vi "IDS_ecu_getParameters.vi"(8 "error in (no error)":errorcluster, 11 "deviceHandle":i32) -> (0 "error out":errorcluster, 2 "ECU parameters":T1, 3 "deviceHandle out":i32)   [LabVIEW 2016]
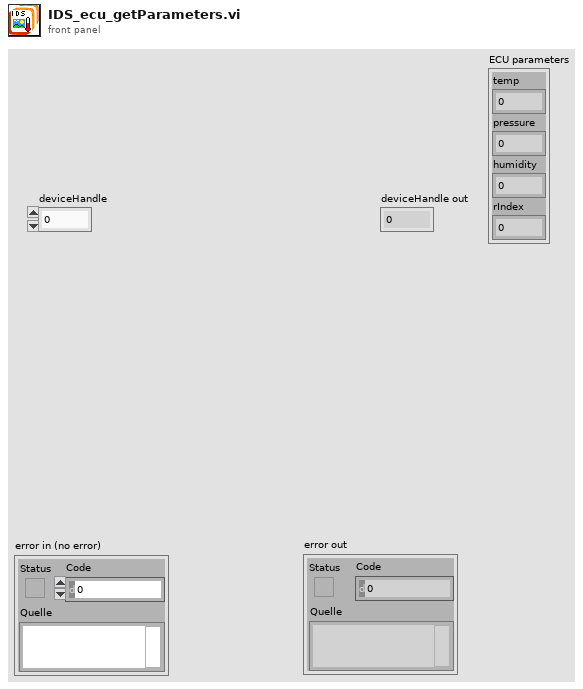
[diagram p1: front panel]
types:
  T1 = cluster{"temp":dbl, "pressure":dbl, "humidity":dbl, "rIndex":dbl}
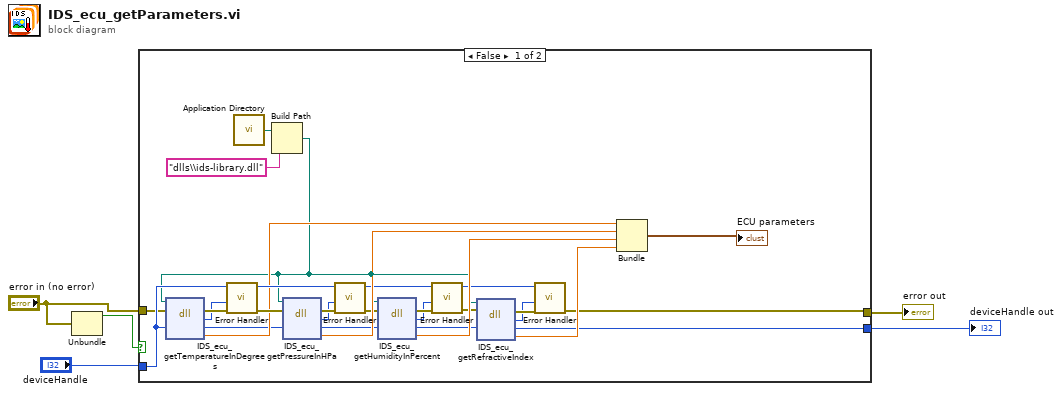
[diagram p0: block diagram]
diagram:
  n1 = Unbundle("error in (no error)") -> ("status"=w2:bool)  [unwired: 2 out]
  n2 = case shown="False" w2 {
    tunnel: [w10 w36] -> w5
    tunnel: [w11 w35] -> w4
    tunnel: "deviceHandle" -> [w20 w35]
    tunnel: "error in (no error)" -> [w14 w36]
    frame False {
      n3 = call <vilib>:"Application Directory.vi"() -> ("Application Directory"=w8:path)
      n4 = Build Path(base path=w8, name or relative path="dlls\\ids-library.dll" ("ipAddress")) -> (appended path=w6:path)
      n5 = dll-call lib="C:/Users/matheus/Desktop/LabVIEW_Draft_V1.6.0/dlls/ids-library.*" fn="IDS_ecu_getTemperatureInDegrees"(path in=w6, error in=w14, "deviceHandle"=w20) -> (error out=w31:errorcluster, "return type"=w24:i32, "deviceHandle"=w12:i32, "temp"=w13:dbl)  [unwired: 2 in, 1 out]
      n6 = call "Error Handler.vi"("error in (no error)"=w31, "error code"=w24, "deviceHandle"=w20) -> ("error out"=w30:errorcluster, "deviceHandle Out"=w17:i32)  [unwired: 7 in]
      n7 = dll-call lib="C:/Users/matheus/Desktop/LabVIEW_Draft_V1.6.0/dlls/ids-library.*" fn="IDS_ecu_getPressureInHPa"(path in=w6, error in=w30, "deviceHandle"=w12) -> (error out=w29:errorcluster, "return type"=w23:i32, "deviceHandle"=w19:i32, "pressure"=w34:dbl)  [unwired: 2 in, 1 out]
      n8 = call "Error Handler.vi"("error in (no error)"=w29, "error code"=w23, "deviceHandle"=w17) -> ("error out"=w28:errorcluster, "deviceHandle Out"=w16:i32)  [unwired: 7 in]
      n9 = dll-call lib="C:/Users/matheus/Desktop/LabVIEW_Draft_V1.6.0/dlls/ids-library.*" fn="IDS_ecu_getHumidityInPercent"(path in=w6, error in=w28, "deviceHandle"=w19) -> (error out=w27:errorcluster, "return type"=w22:i32, "deviceHandle"=w18:i32, "humidity"=w33:dbl)  [unwired: 2 in, 1 out]
      n10 = call "Error Handler.vi"("error in (no error)"=w27, "error code"=w22, "deviceHandle"=w16) -> ("error out"=w26:errorcluster, "deviceHandle Out"=w15:i32)  [unwired: 7 in]
      n11 = dll-call lib="C:/Users/matheus/Desktop/LabVIEW_Draft_V1.6.0/dlls/ids-library.*" fn="IDS_ecu_getRefractiveIndex"(path in=w6, error in=w26, "deviceHandle"=w18) -> (error out=w25:errorcluster, "return type"=w21:i32, "deviceHandle"=w11:i32, "rIndex"=w32:dbl)  [unwired: 2 in, 1 out]
      n12 = call "Error Handler.vi"("error in (no error)"=w25, "error code"=w21, "deviceHandle"=w15) -> ("error out"=w10:errorcluster)  [unwired: 7 in, 1 out]
      n13 = Bundle("temp"=w13, "pressure"=w34, "humidity"=w33, "rIndex"=w32) -> (→"ECU parameters":T1)  [unwired: 1 in]
    }
    frame True {
    }
  }
  "error out" <- w5
  "deviceHandle out" <- w4
